vi "Ricalcola Vn In.vi"(7 "id":i32, 9 "In [A]":dbl, 11 "Vn [V]":dbl) -> (1 "In out":dbl, 3 "Vn out":dbl)   [LabVIEW 2019]
panel:
  out "appended array":bool[](array[boolean])
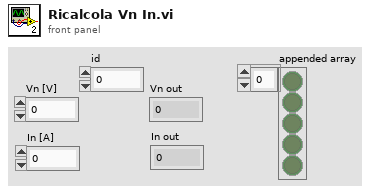
[diagram p1: front panel]
types:
  T1 = enum32{"No Selection", "INVERTER 1 [7,5kW]", "INVERTER 2 [75kW]", "INVERTER 3"}
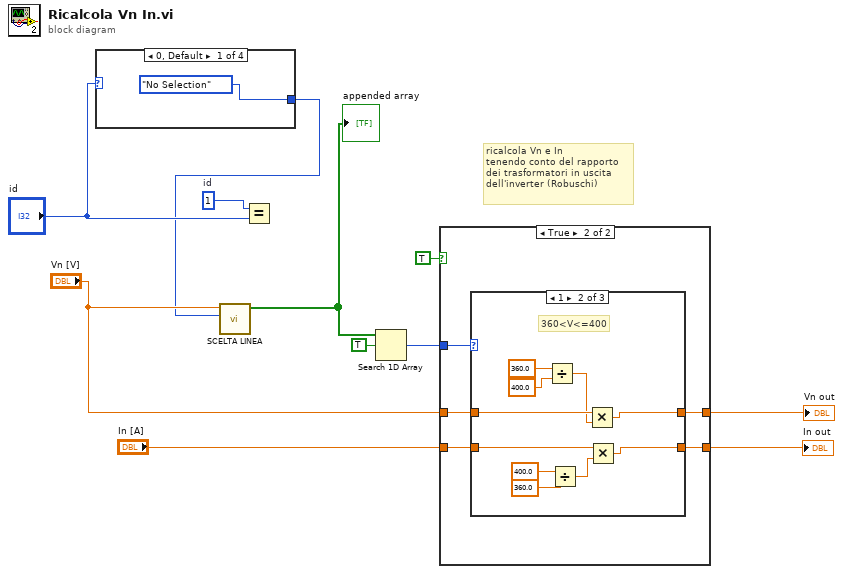
[diagram p0: block diagram]
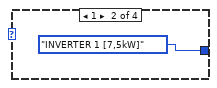
[diagram p2: hidden frame]
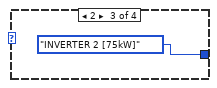
[diagram p3: hidden frame]
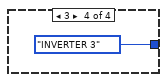
[diagram p4: hidden frame]
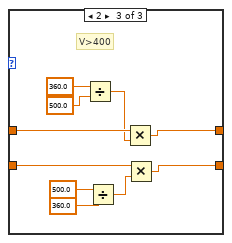
[diagram p7: hidden frame]
diagram:
  w8 = 1  # id
  # "ricalcola Vn e In\ntenendo conto del rapporto\ndei trasformatori in uscita\ndell'inverter (Robuschi)"
  n1 = case shown="0, Default" "id" {
    tunnel: [T1."No Selection" ("Scelta inverter") T1."INVERTER 1 [7,5kW]" ("Scelta inverter") T1."INVERTER 2 [75kW]" ("Scelta inverter") T1."INVERTER 3" ("Scelta inverter")] -> w1
    frame 0, Default {
    }
    frame 1 {
    }
    frame 2 {
    }
    frame 3 {
    }
  }
  n2 = call "SCELTA LINEA.vi"("Scelta inverter"=w1, "Vn [V]"="Vn [V]") -> ("Array"=w11:bool[])  [unwired: 9 in]
  "appended array" <- w11
  n3 = Equal?(x=w8, y="id") -> ()  [unwired: 1 out]
  n4 = Search 1D Array(1D array=w11, element=TRUE) -> (index of element=w9:i32)  [unwired: 1 in]
  n5 = case shown="True" TRUE {
    tunnel: w9 -> [_ w22]
    tunnel: [w17 w21] -> w4
    tunnel: "Vn [V]" -> [w17 w20]
    tunnel: [w16 w19] -> w3
    tunnel: "In [A]" -> [w16 w18]
    frame False {
    }
    frame True {
      n6 = case shown="1" w22 {
        tunnel: [w24 w29 w39] -> w21
        tunnel: w20 -> [w24 w34 w44]
        tunnel: [w23 w28 w38] -> w19
        tunnel: w18 -> [w23 w30 w40]
        frame 0, Default {
          # "V <= 360V"
        }
        frame 1 {
          # "360<V<=400"
          n7 = Divide(x=360.0, y=400.0) -> (x/y=w33:dbl)
          n8 = Divide(x=400.0, y=360.0) -> (x/y=w25:dbl)
          n9 = Multiply(x=w34, y=w33) -> (x*y=w29:dbl)
          n10 = Multiply(x=w30, y=w25) -> (x*y=w28:dbl)
        }
        frame 2 {
          # "V>400"
          n11 = Divide(x=360.0, y=500.0) -> (x/y=w43:dbl)
          n12 = Divide(x=500.0, y=360.0) -> (x/y=w35:dbl)
          n13 = Multiply(x=w44, y=w43) -> (x*y=w39:dbl)
          n14 = Multiply(x=w40, y=w35) -> (x*y=w38:dbl)
        }
      }
    }
  }
  "Vn out" <- w4
  "In out" <- w3
